vi "GFITS_IsTestImage.vi"(10 "Database RefNum in":T1) -> (1 "forcedfits?":bool, 2 "testonly":bool)   [LabVIEW 2016]
uses:
  DBSHAND/private/vis/DatabaseHand_RefNum.ctl
  DBSHAND/private/vis/DatabaseHand_Element_Get(bool).vi
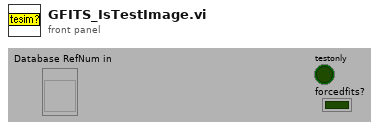
[diagram p1: front panel]
types:
  T1 = typedef "DatabaseHand_RefNum.ctl" = refnum<vi>
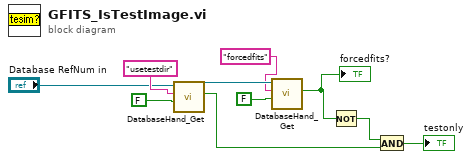
[diagram p0: block diagram]
diagram:
  n1 = call-poly "DatabaseHand_Get.vi"("default value"=FALSE, "name"="usetestdir", "Database RefNum in"="Database RefNum in") -> ("value"=w3:bool, "Database RefNum out"=w7:T1)  [unwired: 2 in, 5 out]
  n2 = call-poly "DatabaseHand_Get.vi"("default value"=FALSE, "name"="forcedfits", "Database RefNum in"=w7) -> ("value"=w1:bool)  [unwired: 2 in, 6 out]
  "forcedfits?" <- w1
  n3 = Not(x=w1) -> (.not. x?=w4:bool)
  n4 = And(x=w4, y=w3) -> (x .and. y?=→"testonly":bool)
